vi "Execute Add RefNum to Actor Data.vi"(6 "Mouse Position":T1, 8 "User VI Ref":refnum<vi>, 9 "Menu Item Tag Suffix":string, 10 "Remaining Items":refnum<vi>[](array[refnum]), 11 "Affected Items":T2) -> (0 "Fail transaction?":bool)   [LabVIEW 2020]
doc: "This VI is part of a plug-in for modifying the LabVIEW shortcut menus. This is the execute VI which is called when the shortcut menu is chosen by the user. It performs the action of the selected menu item."
uses:
  Add RefNum to Actor Data.ctl
  <vilib>/Utility/miscctls.llb/LVPositionTypeDef.ctl
panel:
  # "All controls on this panel except \"Affected Items\" have been locked to prevent accidental edits. Changing the control names or types, other than the elements of the \"Affected Items\" cluster will make the VI unusable as a menu plugin.\n\nSee Context Help for each control for details about its use."
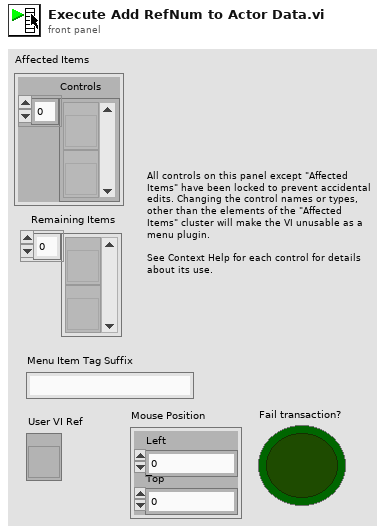
[diagram p1: front panel]
types:
  T1 = typedef "LVPositionTypeDef.ctl" = cluster{"Left":i32, "Top":i32}
  T2 = typedef "Add RefNum to Actor Data.ctl" = cluster{"Controls":refnum<vi>[]}
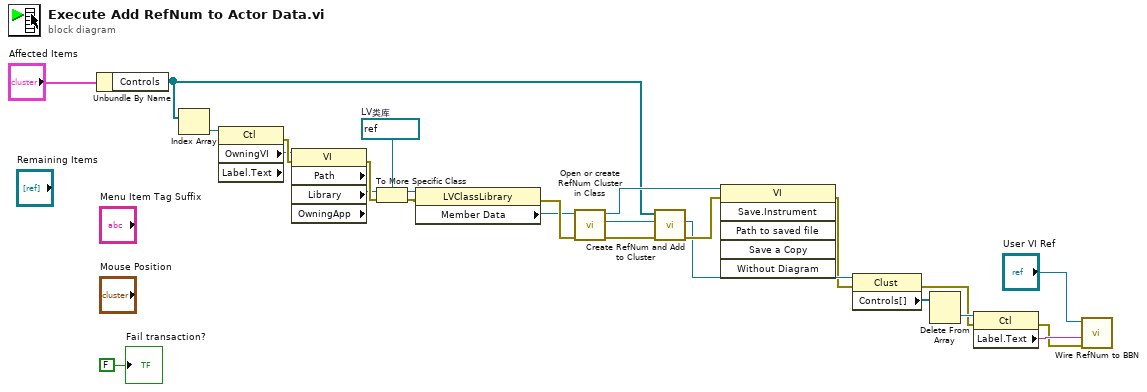
[diagram p0: block diagram]
diagram:
  w15 = refnum<vi> refnum  # LV类库
  n1 = Unbundle By Name("Affected Items") -> ("Controls"=w4:refnum<vi>[])
  n2 = Index Array(array=w4) -> (element=w9:refnum<vi>)  [unwired: 1 in]
  n3 = property class="Ctl" props=["OwningVI", "Label", "Text"](reference=w9) -> (error out=w25:errorcluster, "OwningVI"=w17:refnum<vi>)  [unwired: 1 in, 2 out]
  n4 = property class="VI" props=["Path", "Library", "OwningApp"](reference=w17, error in=w25) -> (error out=w23:errorcluster, "Library"=w16:refnum<vi>)  [unwired: 3 out]
  n5 = To More Specific Class(target class=w15, reference=w16, error in=w23) -> (specific class reference=w14:refnum<vi>, error out=w24:errorcluster)
  n6 = property class="LVClassLibrary"(reference=w14, error in=w24) -> (error out=w22:errorcluster, "Member Data"=w13:refnum<vi>)  [unwired: 1 out]
  n7 = call "Open or create RefNum Cluster in Class.vi"("error in (no error)"=w22, "VI in"=w13) -> ("error out"=w20:errorcluster, "Cluster out"=w6:refnum<vi>, "VI dub"=w7:refnum<vi>)  [unwired: 7 in]
  n8 = call "Create RefNum and Add to Cluster.vi"("error in (no error)"=w20, "Owning Cluster in"=w6, "Controls"=w4) -> ("error out"=w21:errorcluster, "Owning Cluster out"=w5:refnum<vi>)  [unwired: 6 in, 1 out]
  n9 = invoke class="VI" method="Save.Instrument"(reference=w7, error in=w21) -> (error out=w3:errorcluster)  [unwired: 4 in, 5 out]
  n10 = property class="Clust"(reference=w5, error in=w3) -> (error out=w2:errorcluster, "Controls[]"=w12:refnum<vi>[])  [unwired: 1 out]
  n11 = Delete From Array(array=w12) -> (deleted portion=w11:refnum<vi>)  [unwired: 2 in, 1 out]
  n12 = property class="Ctl"(reference=w11, error in=w2) -> (error out=w1:errorcluster, "Label.Text"=w10:string)  [unwired: 1 out]
  n13 = call "Wire RefNum to BBN.vi"("error in (no error)"=w1, "Label.Text"=w10, "VI in"="User VI Ref") -> ()  [unwired: 8 in, 1 out]
  "Fail transaction?" <- FALSE ("Fail transaction?")
